vi "Write shared variable.vi"(9 "DATO DBL":dbl, 10 "nome shared variable":string) -> (0 "error out":errorcluster)   [LabVIEW 2019]
uses:
  Global IP address server.vi
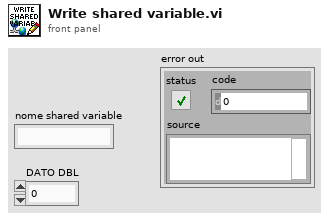
[diagram p1: front panel]
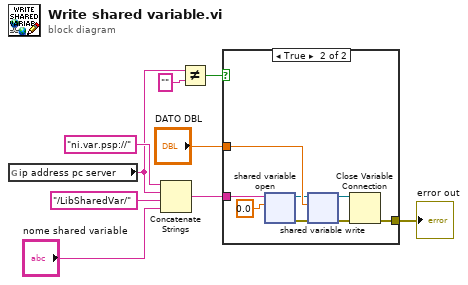
[diagram p0: block diagram]
diagram:
  n1 = global read "Global IP address server.vi" "ip address pc server"() -> (w3:string)
  n2 = Concatenate Strings("ni.var.psp://", w3, "/LibSharedVar/", "nome shared variable") -> (w8:string)
  n3 = Not Equal?(x=w3, y="") -> (x != y?=w1:bool)
  n4 = case shown="True" w1 {
    tunnel: [_ w17] -> w9
    tunnel: w8 -> [_ w14]
    tunnel: "DATO DBL" -> [_ w12]
    frame False {
    }
    frame True {
      n5 = shared-variable-open(w14, 0.0) -> (w10:refnum<k21>, w15:errorcluster)  [unwired: 2 in]
      n6 = shared-variable-write(w10, w15, w12) -> (w13:refnum<k21>, w16:errorcluster)
      n7 = Close Variable Connection(8:w16, 11:w13) -> (0:w17:errorcluster)
    }
  }
  "error out" <- w9
